vi "Write Return Current Status Msg.vi"(10 "EMS Generic Actor.lvlib:Return String Msg.lvclass":refnum<class "Return String Msg.lvclass">, 11 "EMS Generic in":refnum<class "EMS Generic.lvclass">) -> (3 "EMS Generic out":refnum<class "EMS Generic.lvclass">)   [LabVIEW 2018, in "EMS Generic Actor.lvlib" / "EMS Generic.lvclass"]
uses:
  EMS Generic.lvclass
  EMS Generic Messages/Return String Msg/Return String Msg.lvclass
  EMS Generic.lvclass/EMS Generic.ctl
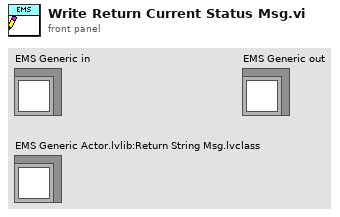
[diagram p1: front panel]
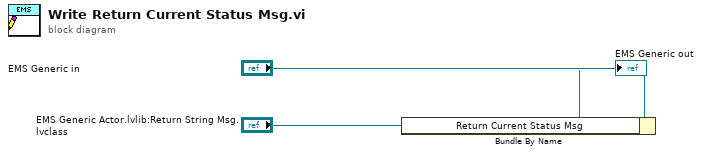
[diagram p0: block diagram]
diagram:
  n1 = Bundle By Name(cluster="EMS Generic in", "Return Current Status Msg"="EMS Generic Actor.lvlib:Return String Msg.lvclass") -> (→"EMS Generic out":refnum<class "EMS Generic.lvclass">)
